vi "rotate bitstream.vi"(10 "QAM system parameters":T1, 11 "input bit stream":i8[](array[numeric])) -> (2 "output bit stream rotated using QAM parameters":i8[](array[numeric]), 3 "output bit stream rotated M-ary 4":i8[](array[numeric]))   [LabVIEW 2013]
panel:
  out "z*i":cdb[](array[numeric])
  out "z":cdb[](array[numeric])
  out "Array 2":i32[](array[numeric])
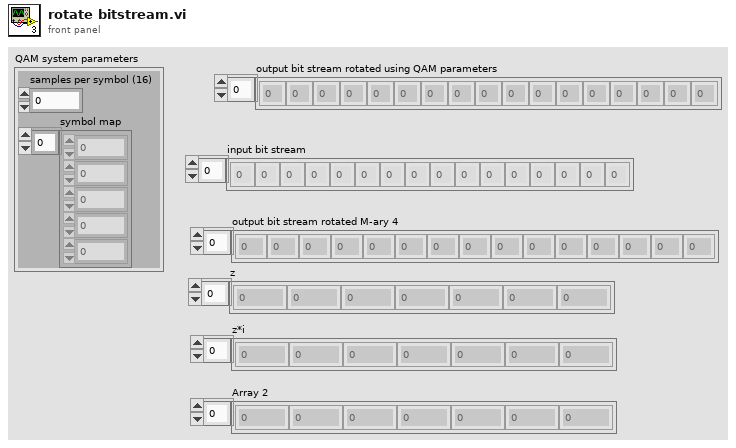
[diagram p1: front panel]
types:
  T1 = cluster{"samples per symbol (16)":i32, "symbol map":cdb[]}
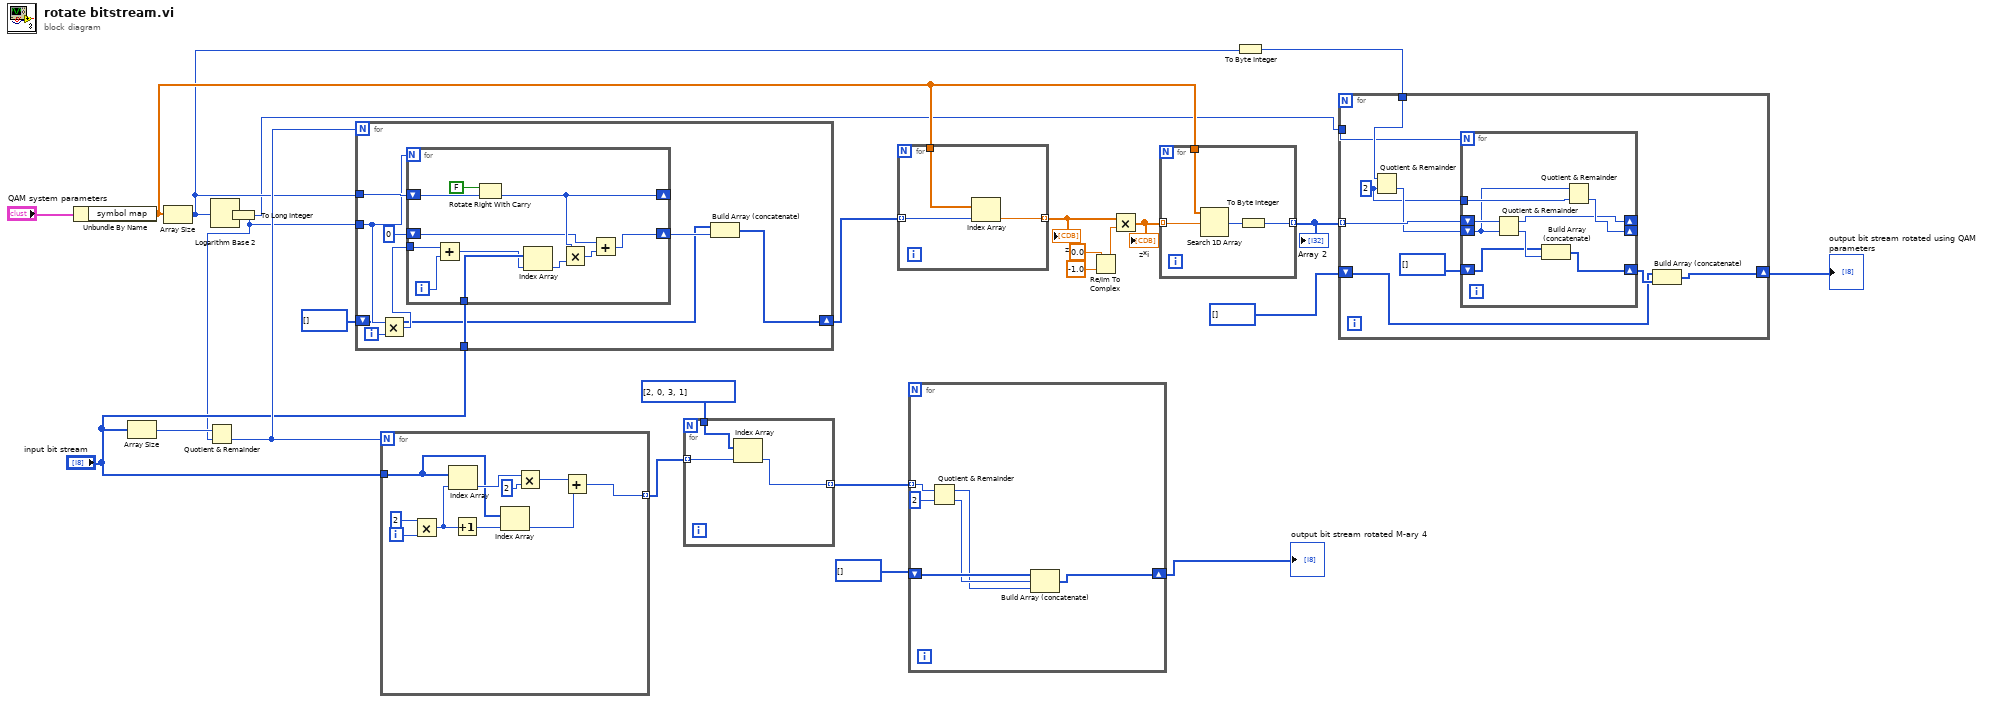
[diagram p0: block diagram]
diagram:
  n1 = Unbundle By Name("QAM system parameters") -> ("symbol map"=w7:cdb[])
  n2 = Array Size(array="input bit stream") -> (size(s)=w24:i32)
  n3 = Array Size(array=w7) -> (size(s)=w3:i32)
  n4 = Logarithm Base 2(1:w3) -> (0:w17:dbl)
  n5 = To Long Integer(number=w17) -> (32bit integer=w2:i32)
  n6 = Quotient & Remainder(x=w24, y=w2) -> (floor(x/y)=w16:i32)  [unwired: 1 out]
  n7 = for {
    N: w16 -> [_]
    tunnel: w2 -> [w31]
    tunnel: w3 -> [w33]
    tunnel: "input bit stream" -> [w29]
    shift-right: [w27] -> w13
    shift-left: i32[] [] -> [w25]
    i -> [w32]
    n8 = Multiply(x=w31, y=w32) -> (x*y=w30:i32)
    n9 = for {
      N: w31 -> [_]
      shift-right: [w38] -> _
      shift-left: w33 -> [w44]
      tunnel: w30 -> [w43]
      tunnel: w29 -> [w41]
      shift-right: [w35] -> w26
      shift-left: 0 -> [w36]
      i -> [w42]
      n10 = Add(x=w43, y=w42) -> (x+y=w40:i32)
      n11 = Rotate Right With Carry(2:w44, 3:FALSE ("carry")) -> (0:w38:i32)  [unwired: 1 out]
      n12 = Index Array(array=w41, index=w40) -> (element=w39:i8)
      n13 = Multiply(x=w38, y=w39) -> (x*y=w37:i32)
      n14 = Add(x=w36, y=w37) -> (x+y=w35:i32)
    }
    n15 = Build Array (concatenate)(w25, w26) -> (w27:i32[])
  }
  n16 = for {
    N: w16 -> [_]
    tunnel: "input bit stream" -> [w48]
    tunnel: [w45] -> w20 mode=indexing
    i -> [w54]
    n17 = Multiply(x=2, y=w54) -> (x*y=w50:i32)
    n18 = Index Array(array=w48, index=w50) -> (element=w52:i8)
    n19 = Increment(x=w50) -> (x+1=w49:i32)
    n20 = Index Array(array=w48, index=w49) -> (element=w47:i8)
    n21 = Multiply(x=w52, y=i8 2) -> (x*y=w46:i8)
    n22 = Add(x=w46, y=w47) -> (x+y=w45:i8)
  }
  n23 = for {
    tunnel: i8[] [2, 0, 3, 1] -> [w57]
    tunnel: w20 -> [w56] mode=indexing
    tunnel: [w55] -> w19 mode=indexing
    n24 = Index Array(array=w57, index=w56) -> (element=w55:i8)
  }
  n25 = for {
    tunnel: w7 -> [w60]
    tunnel: w13 -> [w59] mode=indexing
    tunnel: [w58] -> w12 mode=indexing
    n26 = Index Array(array=w60, index=w59) -> (element=w58:cdb)
  }
  "z" <- w12
  n27 = for {
    tunnel: w19 -> [w65] mode=indexing
    shift-right: [w61] -> w22
    shift-left: i8[] [] ("output bit stream") -> [w66]
    n28 = Quotient & Remainder(x=w65, y=i8 2) -> (x-y*floor(x/y)=w62:i8, floor(x/y)=w63:i8)
    n29 = Build Array (concatenate)(w66, w63, w62) -> (w61:i8[])
  }
  "output bit stream rotated M-ary 4" <- w22
  n30 = Re/Im To Complex(1:-1.0 ("y"), 2:0.0 ("x")) -> (0:w9:cdb)
  n31 = Multiply(x=w12, y=w9) -> (x*y=w8:cdb[])
  "z*i" <- w8
  n32 = for {
    tunnel: w8 -> [w69] mode=indexing
    tunnel: w7 -> [w70]
    tunnel: [w67] -> w6 mode=indexing
    n33 = Search 1D Array(1D array=w70, element=w69) -> (index of element=w68:i32)  [unwired: 1 in]
    n34 = To Byte Integer(number=w68) -> (8bit integer=w67:i8)
  }
  "Array 2" <- w6
  n35 = To Byte Integer(number=w3) -> (8bit integer=w1:i8)
  n36 = for {
    tunnel: w6 -> [w79] mode=indexing
    tunnel: w1 -> [w78]
    shift-right: [w74] -> w4
    shift-left: i8[] [] -> [w73]
    tunnel: w2 -> [w71]
    w76 = i8 2 ("y")
    n37 = Quotient & Remainder(x=w78, y=w76) -> (floor(x/y)=w77:i8)  [unwired: 1 out]
    n38 = for {
      N: w71 -> [_]
      shift-right: [w86] -> w75
      shift-left: i8[] [] -> [w85]
      shift-right: [w81] -> _
      shift-left: w77 -> [w82]
      tunnel: w76 -> [w84]
      shift-right: [w80] -> _
      shift-left: w79 -> [w83]
      n39 = Quotient & Remainder(x=w83, y=w82) -> (x-y*floor(x/y)=w80:i8, floor(x/y)=w87:i8)
      n40 = Build Array (concatenate)(w85, w87) -> (w86:i8[])
      n41 = Quotient & Remainder(x=w82, y=w84) -> (floor(x/y)=w81:i8)  [unwired: 1 out]
    }
    n42 = Build Array (concatenate)(w73, w75) -> (w74:i8[])
  }
  "output bit stream rotated using QAM parameters" <- w4
